vi "set_data.vi"(9 "new data":T1, 10 "point to set index":cluster{"Numeric":i32, "Numeric":i32}, 11 "SquareTeam.lvlib:MyTeam.lvclass 2":refnum<class "MyTeam.lvclass">) -> (3 "SquareTeam.lvlib:MyTeam.lvclass":refnum<class "MyTeam.lvclass">)   [LabVIEW 2020, in "The_Hill_Youth.lvlib" / "MyTeam.lvclass"]
uses:
  MyTeam.lvclass
  map_point.ctl
  MyTeam.lvclass/MyTeam.ctl
  The_Hill_Youth.lvlib
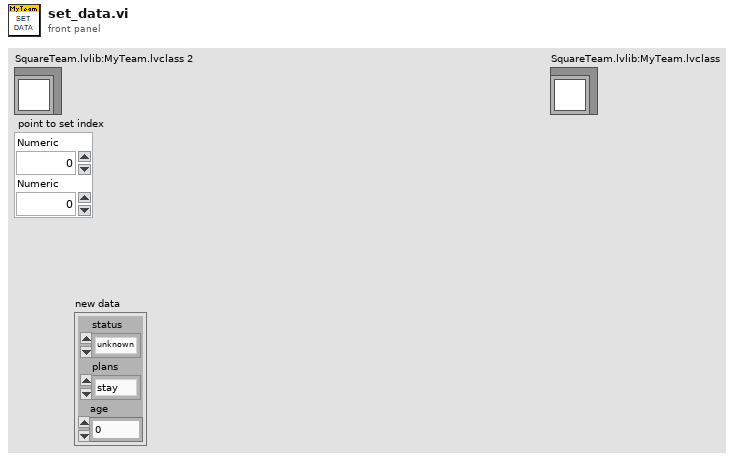
[diagram p1: front panel]
types:
  T1 = typedef "The_Hill_Youth.lvlib/map_point.ctl" = cluster{"status":enum16{"unknown", "frind", "enemy", "empty"}, "plans":enum16{"stay", "duplicate", "attack", "move to", "no plans"}, "age":dbl}
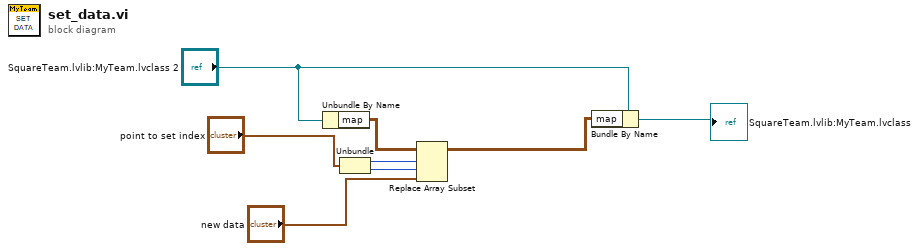
[diagram p0: block diagram]
diagram:
  n1 = Unbundle By Name("SquareTeam.lvlib:MyTeam.lvclass 2") -> ("map"=w6:T1[][])
  n2 = Unbundle("point to set index") -> ("Numeric"=w3:i32, "Numeric"=w2:i32)
  n3 = Replace Array Subset(array=w6, new element="new data", index (row)=w3, index (col)=w2) -> (w5:T1[][])
  n4 = Bundle By Name(cluster="SquareTeam.lvlib:MyTeam.lvclass 2", "map"=w5) -> (→"SquareTeam.lvlib:MyTeam.lvclass":refnum<class "MyTeam.lvclass">)
